vi "GetSpots.vi"(5 "New Image":T1, 6 "Threshold":dbl=20.0 format="%.2f", 7 "error in (no error)":errorcluster) -> (0 "Image Dst Out":T1, 1 "Number of Particles":i32, 2 "Coefficients (2D)":sgl[][](array[numeric]) format="%.2f", 3 "error out":errorcluster, 4 "Color Palette":cluster{u8, u8, u8}[](array[cluster]))   [LabVIEW 2009]
uses:
  <vilib>/vision/Image Controls.llb/IMAQ Image.ctl
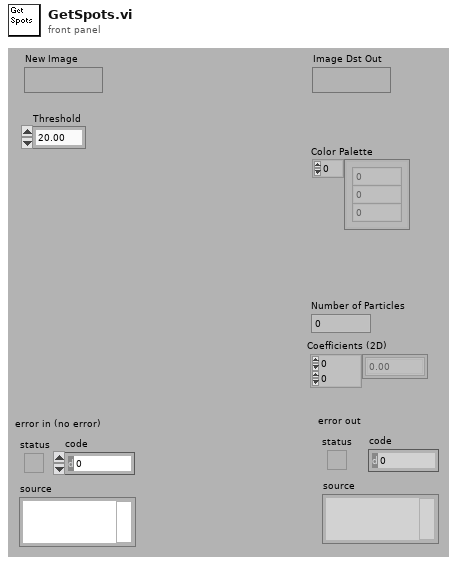
[diagram p1: front panel]
types:
  T1 = typedef "IMAQ Image.ctl" = refnum<image>
  T2 = enum32{"Gray", "Binary", "Gradient", "Rainbow", "Temperature"}
  T3 = cluster{"Parameter":enum32{"Area (pixels)", "Area (calibrated)", "Number of holes", "Holes area (pixels)", "Total area (pixels)", "Scanned area (pixels)", "Ratio Area/Scanned area (%)", "Ratio Area/Total area (%)", "Center of mass (X)", "Center of mass (Y)", "Left column (X)", "Upper row (Y)", "Right column (X)", "Lower row (Y)", "Width (pixels)", "Height (pixels)", "Longest segment length", "Longest segment left column (X)", "Longest segment top row  (Y)", "Perimeter", "Holes perimeter", "SumX", "SumY", "SumXX", "SumYY", "SumXY", "Corrected projection X", "Corrected projection Y", "Moment of inertia Ixx", "Moment of inertia Iyy", "Moment of inertia Ixy", "Mean chord X", "Mean chord Y", "Max intercept", "Mean intercept perpendicular", "Particle orientation", "Equivalent ellipse minor axis", "Ellipse major axis", "Ellipse minor axis", "Ratio of equivalent ellipse axis", "Rectangle big side", "Rectangle small side", "Ratio of equivalent rectangle sides", "Elongation factor", "Compactness factor", "Heywood circularity factor", "Type factor", "Hydraulic radius", "Waddel disk diameter", "Diagonal"}, "Lower Value":sgl, "Upper Value":sgl, "Interval":bool}[]
  T4 = cluster{"Area (pixels)":i32, "Area (calibrated)":sgl, "Perimeter":sgl, "Number of Holes":i32, "Hole's Area (pixels)":i32, "Hole's Perimeter":sgl, "Global Rectangle":cluster{"x1Left":i32, "y1Top":i32, "x2Right":i32, "y2Bottom":i32}, "åx":sgl, "åy":sgl, "åxx":sgl, " åyy":sgl, "åxy":sgl, "Longest Segment Length":i32, "Longest Segment Coordinates":cluster{"x":i32, "y":i32}, "Projection x":i32, "Projection y":i32}[]
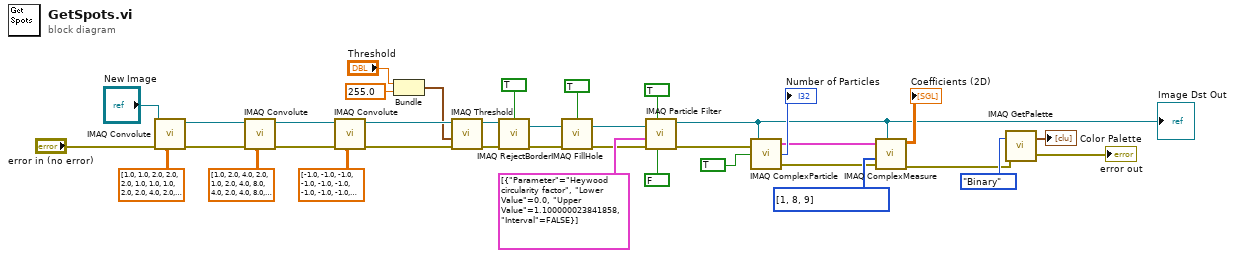
[diagram p0: block diagram]
diagram:
  w19 = i32[] [1, 8, 9] items=["Area (pixels)", "Area (calibrated)", "Number of holes", "Holes area (pixels)", "Total area", "Scanned area", "Ratio Area/Scanned area (%)", "Ratio Area/Total area (%)", "Center of mass (X)", "Center of mass (Y)", "Left column (X)", "Upper row (Y)", "Right column (X)", "Lower row (Y)", "Width", "Height", "Longest segment length", "Longest segment left column (X)", "Longest segment top row  (Y)", "Perimeter", "Hole's perimeter", "SumX", "SumY", "SumXX", "SumYY", "SumXY", "Corrected projection X", "Corrected projection Y", "Moment of inertia Ixx", "Moment of inertia Iyy", "Moment of inertia Ixy", "Mean chord X", "Mean chord Y", "Max intercept", "Mean intercept perpendicular", "Particle orientation", "Equivalent ellipse minor axis", "Ellipse major axis", "Ellipse minor axis", "Ratio of equivalent ellipse axis", "Rectangle big side", "Rectangle small side", "Ratio of equivalent rectangle sides", "Elongation factor", "Compactness factor", "Heywood circularity factor", "Type factor", "Hydraulic radius", "Waddel disk diameter", "Diagonal"] ("Parameters")
  n1 = call "IMAQ Convolute"("Kernel"=sgl[][] [[1.0, 1.0, 2.0, 2.0, 2.0, 1.0, 1.0], [1.0, 2.0, 2.0, 4.0, 2.0, 2.0, 1.0], [2.0, 2.0, 4.0, 8.0, 4.0, 2.0, 2.0], [2.0, 4.0, 8.0, 16.0, 8.0, 4.0, 2.0], [2.0, 2.0, 4.0, 8.0, 4.0, 2.0, 2.0], [1.0, 2.0, 2.0, 4.0, 2.0, 2.0, 1.0], [1.0, 1.0, 2.0, 2.0, 2.0, 1.0, 1.0]], "error in (no error)"="error in (no error)", "Image Src"="New Image") -> ("error out"=w32:errorcluster, "Image Dst Out"=w33:T1)  [unwired: 7 in]
  n2 = call "IMAQ Convolute"("Kernel"=sgl[][] [[1.0, 2.0, 4.0, 2.0, 1.0], [2.0, 4.0, 8.0, 4.0, 2.0], [4.0, 8.0, 16.0, 8.0, 4.0], [2.0, 4.0, 8.0, 4.0, 2.0], [1.0, 2.0, 4.0, 2.0, 1.0]], "error in (no error)"=w32, "Image Src"=w33) -> ("error out"=w29:errorcluster, "Image Dst Out"=w30:T1)  [unwired: 7 in]
  n3 = call "IMAQ Convolute"("Kernel"=sgl[][] [[-1.0, -1.0, -1.0, -1.0, -1.0], [-1.0, -1.0, -1.0, -1.0, -1.0], [-1.0, -1.0, 30.0, -1.0, -1.0], [-1.0, -1.0, -1.0, -1.0, -1.0], [-1.0, -1.0, -1.0, -1.0, -1.0]], "error in (no error)"=w29, "Image Src"=w30) -> ("error out"=w27:errorcluster, "Image Dst Out"=w6:T1)  [unwired: 7 in]
  n4 = Bundle("Threshold"="Threshold", 255.0) -> (w5:cluster{"Threshold":dbl, dbl})  [unwired: 1 in]
  n5 = call "IMAQ Threshold"("Range"=w5, "Image Src"=w6) -> ("Image Dst Out"=w7:T1)  [unwired: 8 in, 1 out]
  n6 = call "IMAQ RejectBorder"("error in (no error)"=w27, "Image Src"=w7, "Connectivity 4/8 (8)"=TRUE) -> ("error out"=w25:errorcluster, "Image Dst Out"=w8:T1)  [unwired: 3 in]
  n7 = call "IMAQ FillHole"("error in (no error)"=w25, "Image Src"=w8, "Connectivity 4/8 (8)"=TRUE) -> ("error out"=w20:errorcluster, "Image Dst Out"=w21:T1)  [unwired: 3 in]
  n8 = call "IMAQ Particle Filter"("Keep/Remove Particles"=FALSE, "Connectivity 4/8 (8)"=TRUE, "error in (no error)"=w20, "Selection Values"=T3 [{"Parameter"=enum."Heywood circularity factor", "Lower Value"=0.0, "Upper Value"=1.1, "Interval"=FALSE}], "Image Src"=w21) -> ("error out"=w13:errorcluster, "Image Dst Out"=w1:T1)  [unwired: 3 in]
  "Image Dst Out" <- w1
  n9 = call "IMAQ ComplexParticle"("error in (no error)"=w13, "Connectivity 4/8 (8)"=TRUE, "Image"=w1) -> ("error out"=w14:errorcluster, "Number of Particles"=→"Number of Particles":i32, "Complex Reports"=w15:T4)
  n10 = call "IMAQ ComplexMeasure"("Image"=w1, "error in (no error)"=w14, "Parameters"=w19, "Complex Reports"=w15) -> ("error out"=w11:errorcluster, "Coefficients (2D)"=→"Coefficients (2D)":sgl[][])  [unwired: 4 in, 2 out]
  n11 = call "IMAQ GetPalette"("Palette Number (gray)"=T2."Binary", "error in (no error)"=w11) -> ("Color Palette"=→"Color Palette":cluster{"Red":u8, "Green":u8, "Blue":u8}[], "error out"=→"error out":errorcluster)  [unwired: 3 in]
